vi "SetCalculationValid.vi"(7 "Name":string, 8 "Working Current":T4, 10 "Features":T2[](array[typedef]), 11 "Type":string) -> (0 "=motor channel":bool, 1 "Motor State":T1, 2 ">min working current":bool, 3 "< max working current":bool)   [LabVIEW 2016, in "McsaAnalysisFunctions.lvlib"]
uses:
  <vilib>/addons/InsightCM/Utilities/Analysis/MCSA/McsaAnalysisFunctions.lvlib
  <vilib>/addons/InsightCM/Utilities/Analysis/MCSA/controls/WorkingCurrent.ctl
  <vilib>/addons/InsightCM/Utilities/Analysis/Shared/controls/Feature.ctl
  <vilib>/addons/InsightCM/Utilities/Analysis/Shared/controls/AmplitudeScale.ctl
  <vilib>/addons/InsightCM/Utilities/Analysis/MCSA/controls/MotorState.ctl
  <vilib>/addons/InsightCM/Utilities/Analysis/Shared/AnalysisHelper.lvlib
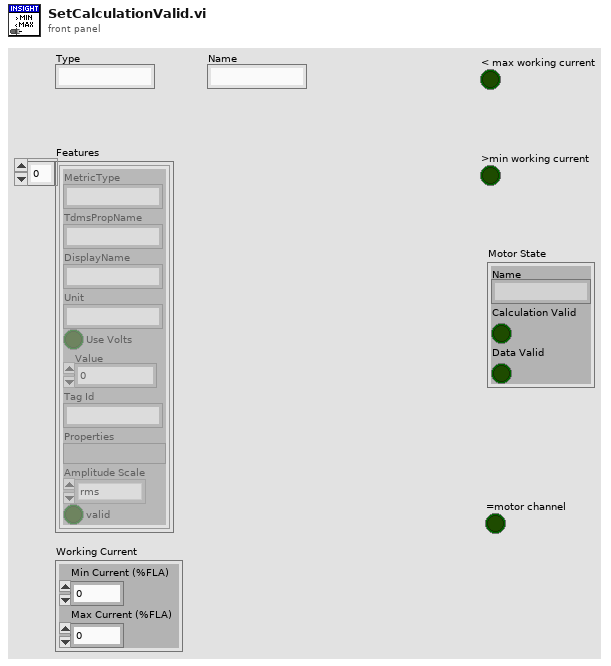
[diagram p1: front panel]
types:
  T1 = typedef "McsaAnalysisFunctions.lvlib/MotorState.ctl" = cluster{"Name":string, "Calculation Valid":bool, "Data Valid":bool}
  T2 = typedef "AnalysisHelper.lvlib/Feature.ctl" = cluster{"MetricType":string, "TdmsPropName":string, "DisplayName":string, "Unit":string, "Use Volts":bool, "Value":dbl, "Tag Id":string, "Properties":variant, "Amplitude Scale":T3, "valid":bool}
  T3 = typedef "AnalysisHelper.lvlib/AmplitudeScale.ctl" = enum16{"rms", "peak", "pk-pk"}
  T4 = typedef "McsaAnalysisFunctions.lvlib/WorkingCurrent.ctl" = cluster{"Min Current (%FLA)":dbl, "Max Current (%FLA)":dbl}
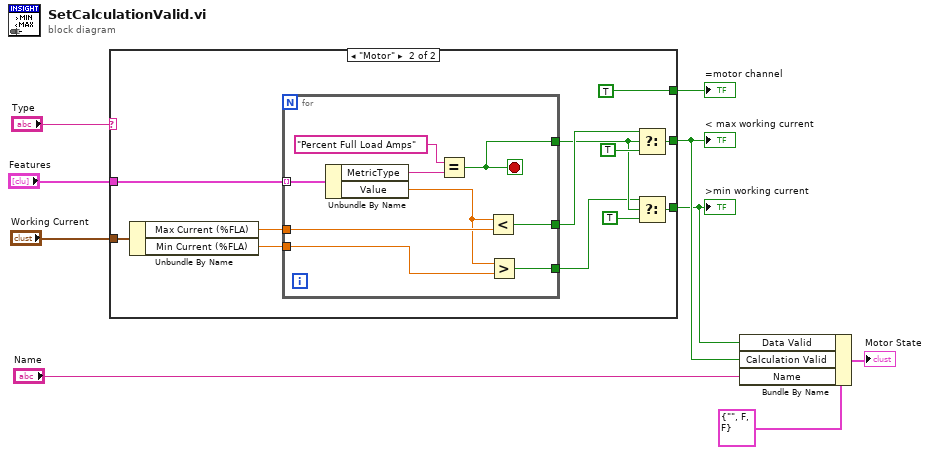
[diagram p0: block diagram]
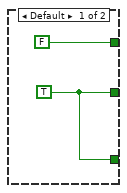
[diagram p2: hidden frame]
diagram:
  n1 = case shown="\"Motor\"" "Type" {
    tunnel: "Working Current" -> [_ w23]
    tunnel: "Features" -> [_ w21]
    tunnel: [w11 w18] -> w2
    tunnel: [w11 w15] -> w1
    tunnel: [FALSE ("f") TRUE ("f")] -> w3
    frame Default {
      w11 = TRUE ("f")
    }
    frame "Motor" {
      n2 = Unbundle By Name(w23) -> ("Max Current (%FLA)"=w22:dbl, "Min Current (%FLA)"=w17:dbl)
      n3 = for {
        tunnel: w22 -> [w32]
        tunnel: w21 -> [w31] mode=indexing
        tunnel: [w28] -> w14
        tunnel: [w27] -> w20
        tunnel: w17 -> [w25]
        tunnel: [w24] -> w13
        stop <- w28 stop-if-true
        n4 = Unbundle By Name(w31) -> ("MetricType"=w30:string, "Value"=w26:dbl)
        n5 = Equal?(x="Percent Full Load Amps", y=w30) -> (x = y?=w28:bool)
        n6 = Less?(x=w26, y=w32) -> (x < y?=w27:bool)
        n7 = Greater?(x=w26, y=w25) -> (0:w24:bool)
      }
      n8 = Select(t=w20, s=w14, f=TRUE) -> (s? t:f=w18:bool)
      n9 = Select(t=w13, s=w14, f=TRUE) -> (s? t:f=w15:bool)
    }
  }
  "< max working current" <- w2
  ">min working current" <- w1
  "=motor channel" <- w3
  n10 = Bundle By Name(cluster=T1 {"Name"="", "Calculation Valid"=FALSE, "Data Valid"=FALSE} ("MCSA FFT"), "Data Valid"=w1, "Calculation Valid"=w2, "Name"="Name") -> (→"Motor State":T1)
